vi "unused_Read selected.vi"(8 "error in (no error)":errorcluster, 11 "GObject in":refnum<class "Generic.lvclass">) -> (0 "error out":errorcluster, 2 "selected":bool, 3 "GObject out":refnum<class "Generic.lvclass">)   [LabVIEW 2023]
uses:
  Generic.lvclass
  Generic.lvclass/Generic.ctl
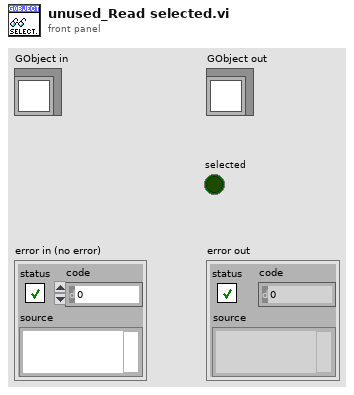
[diagram p1: front panel]
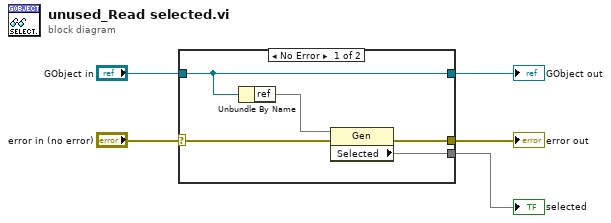
[diagram p0: block diagram]
diagram:
  n1 = case shown="No Error" "error in (no error)" {
    selector: "error in (no error)" -> [w7 w12]
    tunnel: [w6 w12] -> w4
    tunnel: [w10 w11] -> w2
    tunnel: "GObject in" -> [w10 w11]
    tunnel: [w8 _] -> w1
    frame No Error {
      n2 = Unbundle By Name(w10) -> ("ref"=w9)
      n3 = property class="Gen"(reference=w9, error in=w7) -> (error out=w6:errorcluster, "Selected"=w8)  [unwired: 1 out]
    }
    frame Error {
    }
  }
  "error out" <- w4
  "GObject out" <- w2
  "selected" <- w1
